vi "MessageEvents.vi"(9 "Port:":u16=20011, 10 "SSL Vision Address:":string="127.0.0.1", 11 "IA state":T1={"our_robots"=[], "enemy_robots"=[], "balls"=[], "geometry"={"line_width"=0, "field_length"=0, "field_width"=0, "boundary_width"=0, "referee_width"=0, "goal_width"=0, "goal_depth"=0, "goal_wall_width"=0, "center_circle_radius"=0, "defense_radius"=0, "defense_stretch"=0, "free_kick_from_defense_dist"=0, "penalty_spot_from_field_line_dist"=0, "penalty_line_from_spot_dist"=0}, "IA Judge"={"stage"="", "command"="", "our_goalie_id"=0.0, "enemy_goalie_id"=0.0, "command enum"=enum."Halt", "Time"=enum."Azul"}, "Received Timestamp"=timestamp(0 s since 1904-01-01), "Events"={"Touch"=FALSE, "Ball out"=FALSE, "id touch"=0.0, "Ball out of \nVision"=FALSE, "Ball inside \nGoalie area"=FALSE, "Robot not responding"=FALSE, "Robots responding status"=[1.0, 1.0, 1.0, 1.0, 1.0, 1.0], "Enemy Ball \nPossession"=FALSE, "Pass State"=FALSE, "id end of pass"=0.0, "Kick"=FALSE, "Id ini Possession"=0.0, "Ball Possesion"=FALSE, "Id Possesion"=0.0}}) -> (2 "Array":u8[](array[numeric]) format="%02x")   [LabVIEW 2017]
uses:
  Core/AI Input.ctl
  Core/AI Robot.ctl
  Intel/Functions Enum.ctl
  Intel/AttackerStates.ctl
  Core/AI Ball.ctl
  Core/Field Size.ctl
  Core/AI Judge.ctl
  Intel/Command Enum.ctl
  Util/Events/Events.ctl
panel:
  out "error out":errorcluster
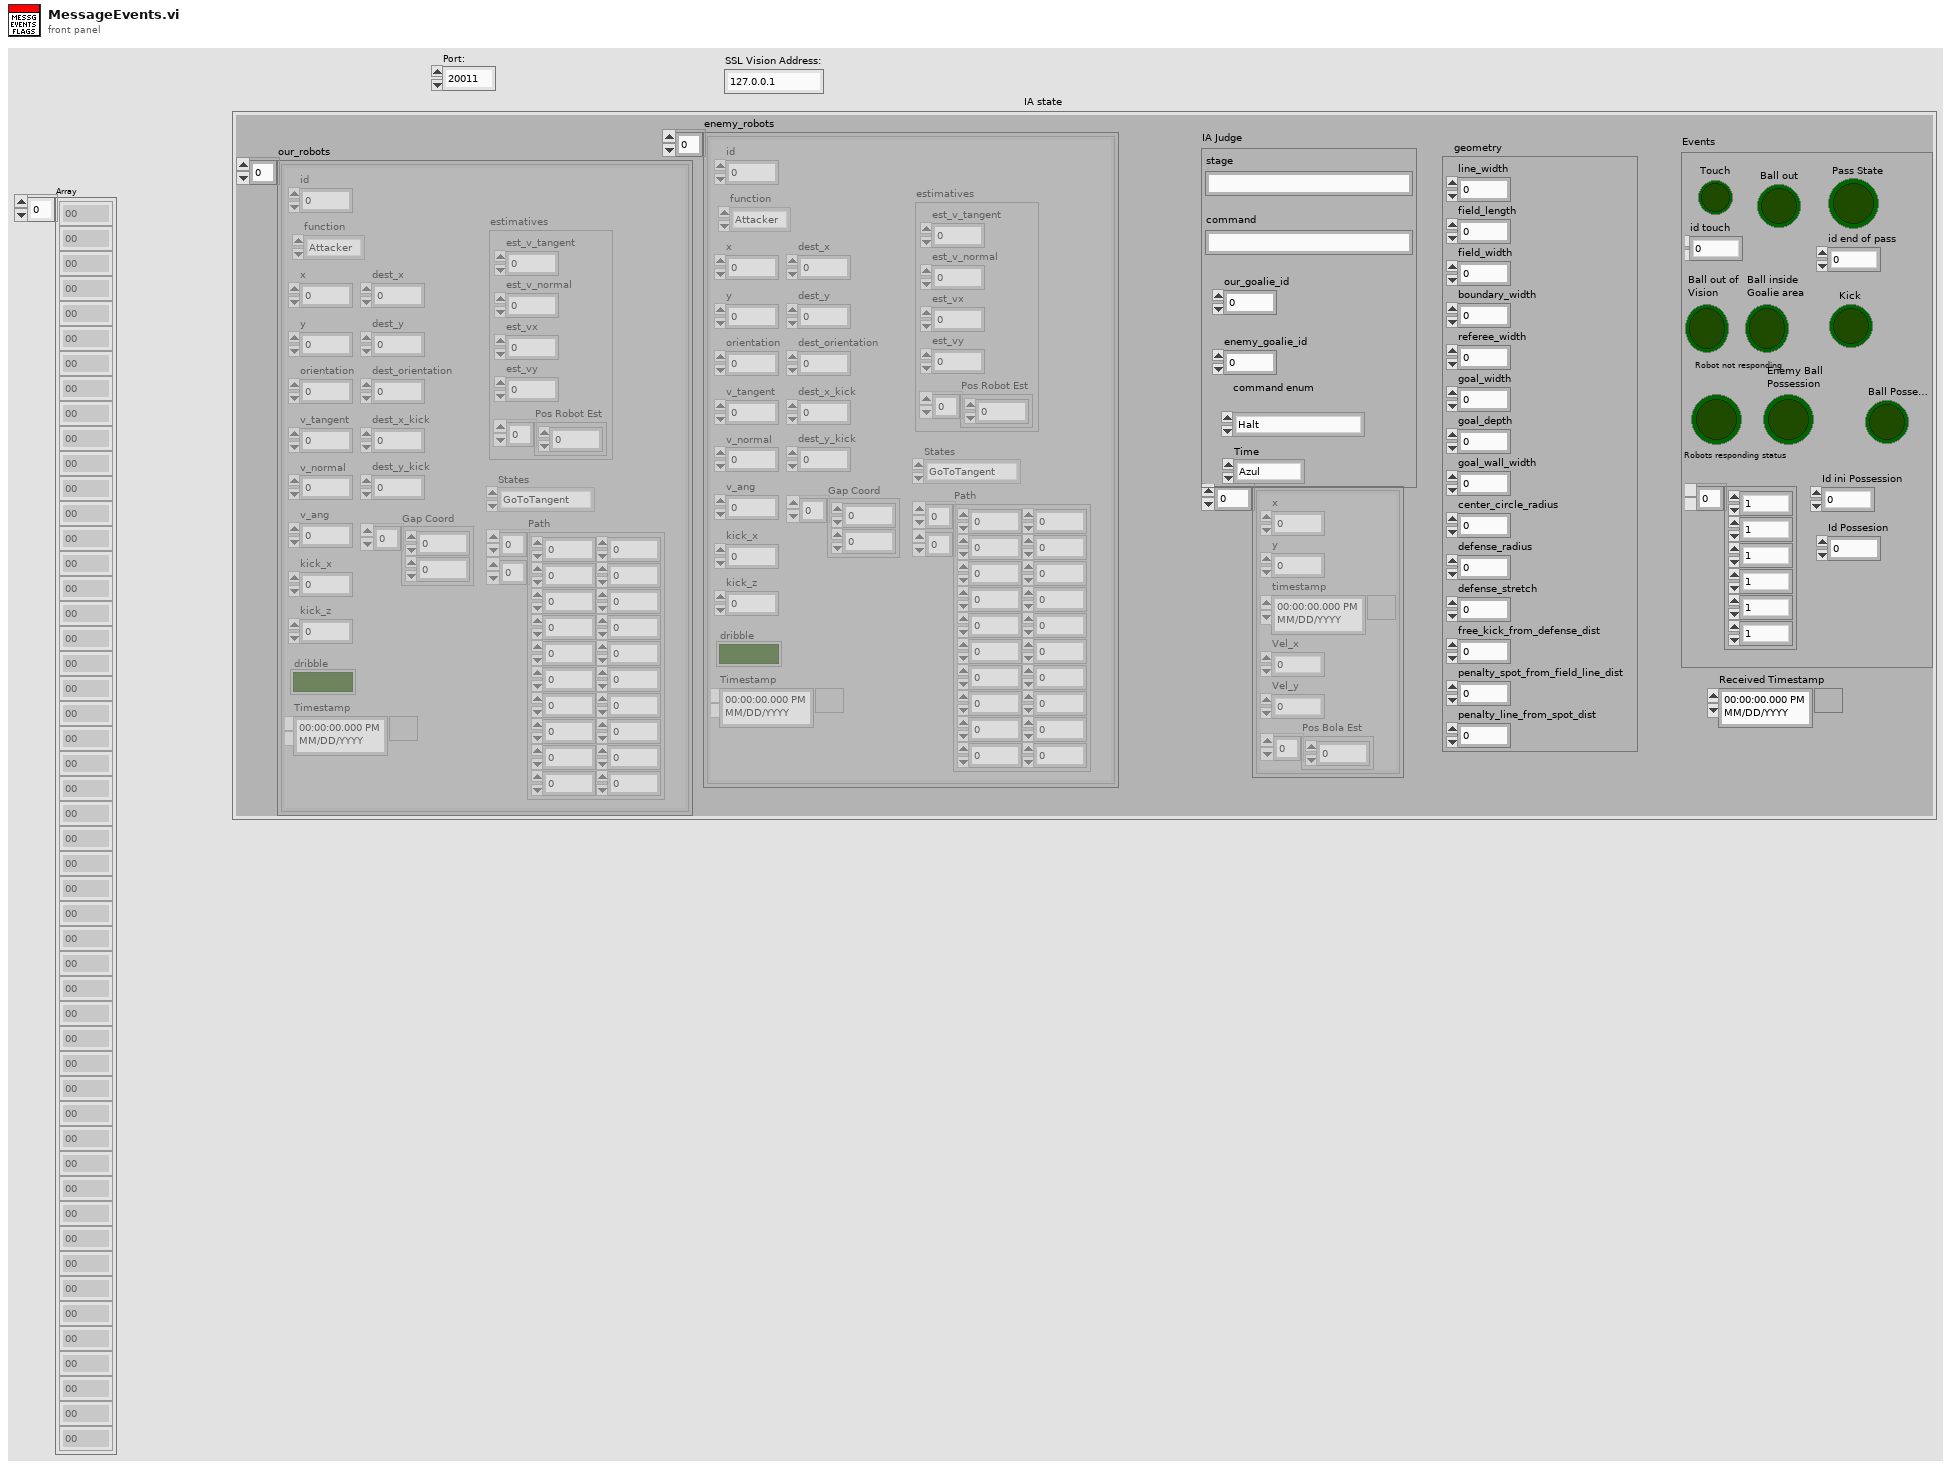
[diagram p1: front panel]
types:
  T1 = typedef "AI Input.ctl" = cluster{"our_robots":T2[], "enemy_robots":T2[], "balls":T5[], "geometry":T6, "IA Judge":T7, "Received Timestamp":timestamp, "Events":T9}
  T2 = typedef "AI Robot.ctl" = cluster{"id":u32, "function":T3, "x":dbl, "y":dbl, "orientation":dbl, "v_tangent":dbl, "v_normal":dbl, "v_ang":dbl, "kick_x":dbl, "kick_z":dbl, "dribble":bool, "Timestamp":timestamp, "dest_x":dbl, "dest_y":dbl, "dest_orientation":dbl, "estimatives":cluster{"est_v_tangent":dbl, "est_v_normal":dbl, "est_vx":dbl, "est_vy":dbl, "Pos Robot Est":dbl[]}, "dest_x_kick":dbl, "dest_y_kick":dbl, "Gap Coord":dbl[], "States":T4, "Path ":dbl[][]}
  T3 = typedef "Functions Enum.ctl" = enum16{"Attacker", "Goalie", "Defender", "Striker", "Goto 0", "Dummy", "Kicker", "ZigZag"}
  T4 = typedef "AttackerStates.ctl" = enum16{"Pass", "GoToTangent", "BallGetting", "GoToKick", ""}
  T5 = typedef "AI Ball.ctl" = cluster{"x":dbl, "y":dbl, "timestamp":timestamp, "Vel_x":dbl, "Vel_y":dbl, "Pos Bola Est":dbl[]}
  T6 = typedef "Field Size.ctl" = cluster{"line_width":u32, "field_length":u32, "field_width":u32, "boundary_width":u32, "referee_width":u32, "goal_width":u32, "goal_depth":u32, "goal_wall_width":u32, "center_circle_radius":u32, "defense_radius":u32, "defense_stretch":u32, "free_kick_from_defense_dist":u32, "penalty_spot_from_field_line_dist":u32, "penalty_line_from_spot_dist":u32}
  T7 = typedef "AI Judge.ctl" = cluster{"stage":string, "command":string, "our_goalie_id":dbl, "enemy_goalie_id":dbl, "command enum":T8, "Time":enum16{"Azul", "Amarelo"}}
  T8 = typedef "Command Enum.ctl" = enum16{"Halt", "Stop", "Force Start", "PKA Normal Start", "Prepare Kickoff Ally", "PKE Normal Start", "Prepare Kickoff Enemy", "Prepare Penalty Ally", "PPA Normal Start", "Prepare Penalty Enemy", "PPE Normal Start", "Direct Free Enemy", "Direct Free Ally", "Indirect Free Enemy", "Indirect Free Ally", "Timeout Enemy", "Timeout Ally", "Goal Enemy", "Goal Ally", "Ball Placement Enemy", "Ball Placement Ally", "Normal Half Time", "Extra Time Break", "Extra Half Time", "None", "Post Game"}
  T9 = typedef "Events.ctl" = cluster{"Touch":bool, "Ball out":bool, "id touch":dbl, "Ball out of \nVision":bool, "Ball inside \nGoalie area":bool, "Robot not responding":bool, "Robots responding status":dbl[], "Enemy Ball \nPossession":bool, "Pass State":bool, "id end of pass":dbl, "Kick":bool, "Id ini Possession":dbl, "Ball Possesion":bool, "Id Possesion":dbl}
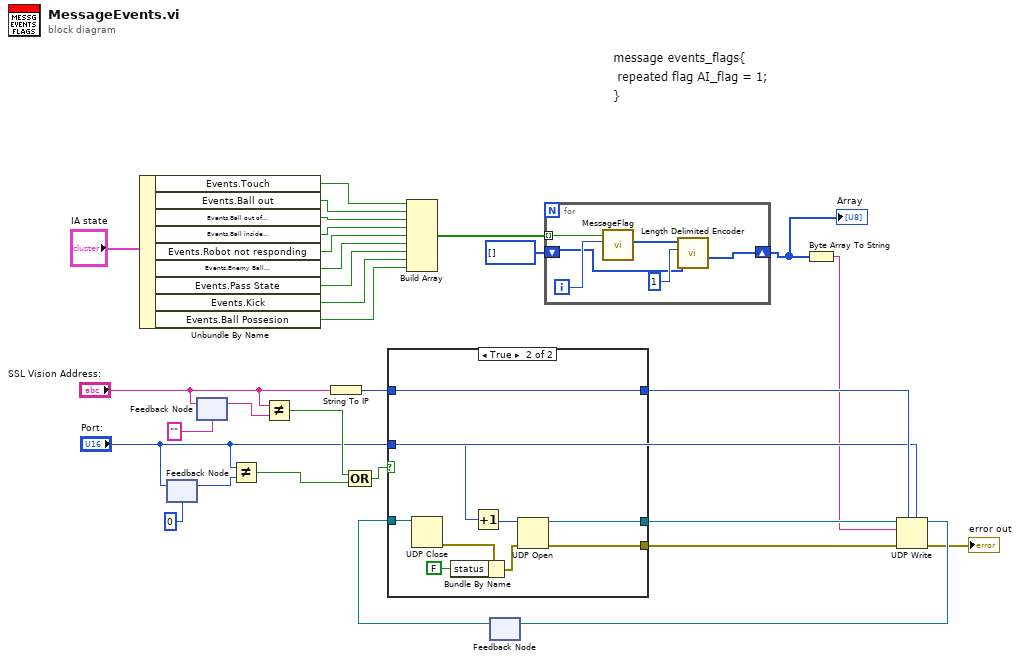
[diagram p0: block diagram]
diagram:
  n1 = Unbundle By Name("IA state") -> ("Events.Touch"=w12:bool, "Events.Ball out"=w11:bool, "Events.Ball out of \nVision"=w10:bool, "Events.Ball inside \nGoalie area"=w9:bool, "Events.Robot not responding"=w8:bool, "Events.Enemy Ball \nPossession"=w7:bool, "Events.Pass State"=w6:bool, "Events.Kick"=w5:bool, "Events.Ball Possesion"=w4:bool)
  n2 = feedback #1(u16 0 ("Port:")) -> (w16:u16)
  n3 = feedback-in #1("Port:") -> ()
  n4 = feedback #2("" ("SSL Vision Address:")) -> (w18:string)
  n5 = feedback-in #2("SSL Vision Address:") -> ()
  n6 = Not Equal?(x="Port:", y=w16) -> (x != y?=w20:bool)
  n7 = Not Equal?(x="SSL Vision Address:", y=w18) -> (x != y?=w19:bool)
  n8 = String To IP(1:"SSL Vision Address:") -> (0:w29:u32)
  n9 = Compound Arithmetic op=OR(w19, w20) -> (w21:bool)
  n10 = Build Array(w12, w11, w10, w9, w8, w7, w6, w5, w4) -> (w1:bool[])
  n11 = feedback #3() -> (w23:refnum<k16>)  [unwired: 1 in]
  n12 = case shown="True" w21 {
    tunnel: [_ w41] -> w15
    tunnel: [w32 w39] -> w24
    tunnel: "Port:" -> [_ w38]
    tunnel: w29 -> [w31 w36]
    tunnel: w23 -> [w32 w37]
    tunnel: [w31 w36] -> w30
    frame False {
    }
    frame True {
      n13 = UDP Close(connection ID=w37) -> (error out=w35:errorcluster)  [unwired: 1 in, 1 out]
      n14 = Bundle By Name(cluster=w35, "status"=FALSE) -> (w34:errorcluster)
      n15 = Increment(x=w38) -> (x+1=w40:u16)
      n16 = UDP Open(8:w34, 11:w40) -> (port=w39:refnum<k16>, 0:w41:errorcluster)  [unwired: 3 in, 1 out]
    }
  }
  n17 = for {
    tunnel: w1 -> [w47] mode=indexing
    shift-right: [w45] -> w3
    shift-left: u8[] [] ("Array") -> [w43]
    i -> [w46]
    n18 = call "MessageFlag.vi"("Id"=w46, "event"=w47) -> ("Array"=w42:u8[])  [unwired: 9 in]
    n19 = call "Length Delimited Encoder.vi"("Array In"=w43, "Key"=u32 1, "Array In 2"=w42) -> ("Array"=w45:u8[])  [unwired: 8 in]
  }
  "Array" <- w3
  n20 = Byte Array To String(unsigned byte array=w3) -> (string=w13:string)
  n21 = UDP Write(address=w30, port or service name="Port:", connection ID=w24, data in=w13, 8:w15) -> (error out=→"error out":errorcluster, 3:w25:refnum<k16>)  [unwired: 1 in]
  n22 = feedback-in #3(w25) -> ()
